vi "fgv_deque.vi"(7 "cmd":enum16{"ini", "read", "add", "close"}(ring), 8 "error":errorcluster, 11 "start pt":cluster{"x":dbl, "y":dbl}) -> (0 "error out":errorcluster, 3 "queue out":refnum<queue>)   [LabVIEW 2019]
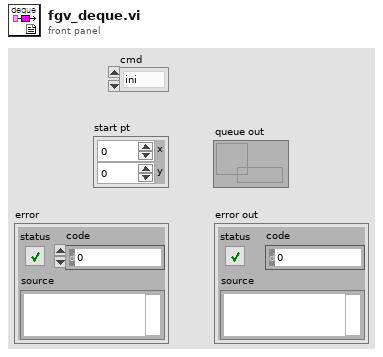
[diagram p1: front panel]
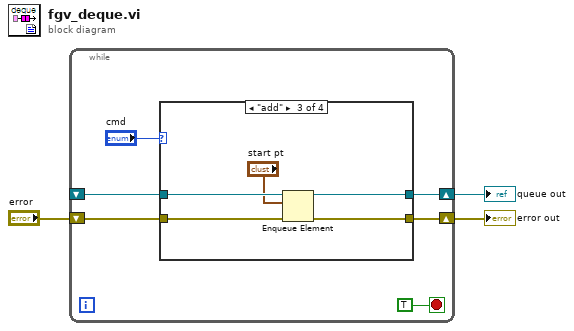
[diagram p0: block diagram]
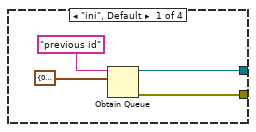
[diagram p2: hidden frame]
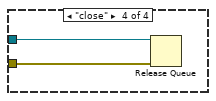
[diagram p4: hidden frame]
diagram:
  n1 = while {
    shift-right: [w6] -> w3
    shift-left: _ -> [w5]
    shift-right: [w7] -> w2
    shift-left: "error" -> [w4]
    stop <- TRUE stop-if-true
    n2 = case shown="\"add\"" "cmd" {
      tunnel: [w13 w14 w17 _] -> w7
      tunnel: [w12 w15 w19 _] -> w6
      tunnel: w5 -> [_ w15 w20 w21]
      tunnel: w4 -> [_ w14 w18 w22]
      frame "ini", Default {
        n3 = Obtain Queue(name (unnamed)="previous id", element data type=cluster{"x":dbl, "y":dbl} {"x"=0.0, "y"=0.0} ("start pt")) -> (queue out=w12:refnum<queue>, error out=w13:errorcluster)  [unwired: 3 in, 1 out]
      }
      frame "read" {
      }
      frame "add" {
        n4 = Enqueue Element(queue=w20, element="start pt", error in (no error)=w18) -> (queue out=w19:refnum<queue>, error out=w17:errorcluster)  [unwired: 1 in, 1 out]
      }
      frame "close" {
        n5 = Release Queue(queue=w21, error in (no error)=w22) -> ()  [unwired: 1 in, 3 out]
      }
    }
  }
  "queue out" <- w3
  "error out" <- w2
